vi "DisplayPathAndPose.vi"(1 "Feed Back Pointing Angle (deg)":dbl, 2 "Feed Back Distance Error (in)":dbl, 3 "Data (index by row)":dbl[][](array[numeric])) -> (0 "Path and Robot Pose":cluster{dbl[], dbl[]}[](graph))   [LabVIEW 2020]
uses:
  Globals/Sensor_Values.vi
panel:
  in  "PID Drive 2":T1(graph)
  in  "PID Heading Indicator":T1(graph)
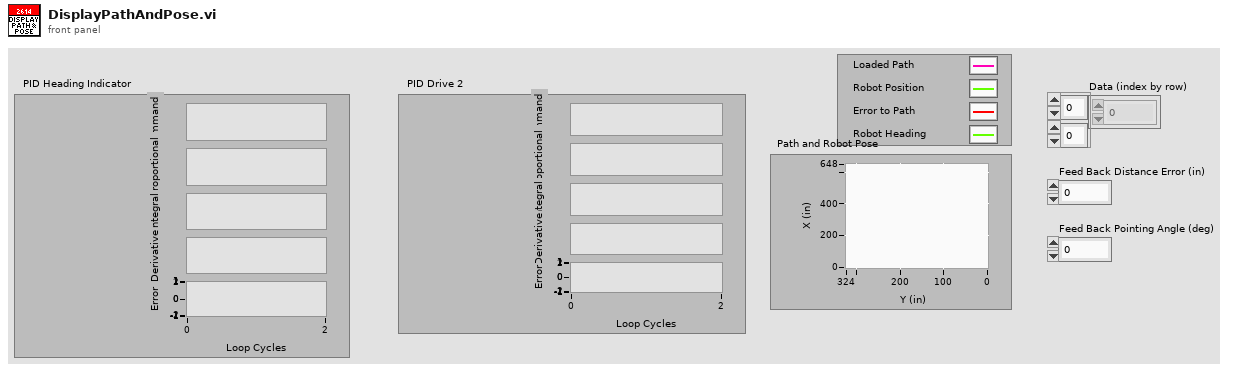
[diagram p1: front panel]
types:
  T1 = cluster{"Command":dbl, "Proportional":dbl, "Integral":dbl, "Derivative":dbl, "Goal":dbl}
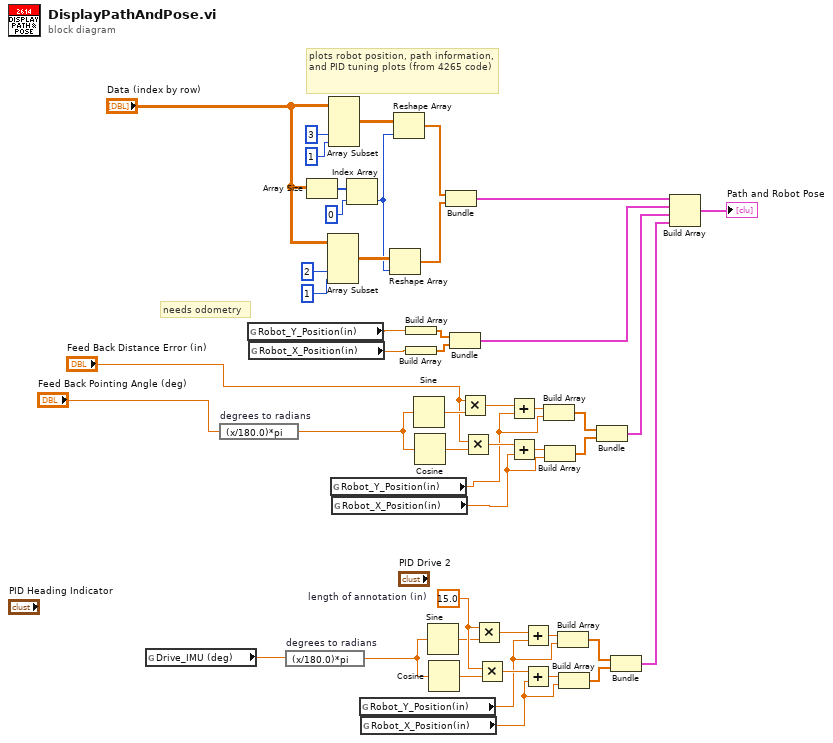
[diagram p0: block diagram]
diagram:
  w43 = 15.0  # length of annotation (in)
  # "needs odometry"
  # "plots robot position, path information, and PID tuning plots (from 4265 code)"
  n1 = global read "Sensor_Values.vi" "Drive_IMU (deg)"() -> (w7:dbl)
  n2 = expression code="(x/180.0)*pi" "degrees to radians"("Feed Back Pointing Angle (deg)") -> (w33:dbl)
  n3 = global read "Sensor_Values.vi" "Robot_Y_Position(in)"() -> (w6:dbl)
  n4 = global read "Sensor_Values.vi" "Robot_X_Position(in)"() -> (w5:dbl)
  n5 = expression code="(x/180.0)*pi" "degrees to radians"(w7) -> (w42:dbl)
  n6 = Array Size(array="Data (index by row)") -> (size(s)=w16:i32[])
  n7 = Array Subset(array="Data (index by row)", index (col)=2 ("index"), length (col)=1 ("length")) -> (w18:dbl[][])  [unwired: 2 in]
  n8 = Array Subset(array="Data (index by row)", index (col)=3 ("index"), length (col)=1 ("length")) -> (w17:dbl[][])  [unwired: 2 in]
  n9 = global read "Sensor_Values.vi" "Robot_Y_Position(in)"() -> (w4:dbl)
  n10 = global read "Sensor_Values.vi" "Robot_X_Position(in)"() -> (w3:dbl)
  n11 = Index Array(array=w16, index=0) -> (element=w15:i32)
  n12 = global read "Sensor_Values.vi" "Robot_Y_Position(in)"() -> (w2:dbl)
  n13 = global read "Sensor_Values.vi" "Robot_X_Position(in)"() -> (w1:dbl)
  n14 = Reshape Array(w18, w15) -> (w46:dbl[])
  n15 = Reshape Array(w17, w15) -> (w45:dbl[])
  n16 = Build Array(w6) -> (w9:dbl[])
  n17 = Build Array(w5) -> (w8:dbl[])
  n18 = Sine(x=w33) -> (sin(x)=w32:dbl)
  n19 = Cosine(x=w33) -> (cos(x)=w31:dbl)
  n20 = Sine(x=w42) -> (sin(x)=w41:dbl)
  n21 = Cosine(x=w42) -> (cos(x)=w40:dbl)
  n22 = Bundle(w45, w46) -> (w13:cluster{dbl[], dbl[]})  [unwired: 1 in]
  n23 = Bundle(w9, w8) -> (w24:cluster{dbl[], dbl[]})  [unwired: 1 in]
  n24 = Multiply(x="Feed Back Distance Error (in)", y=w32) -> (x*y=w30:dbl)
  n25 = Multiply(x="Feed Back Distance Error (in)", y=w31) -> (x*y=w29:dbl)
  n26 = Multiply(x=w43, y=w41) -> (x*y=w39:dbl)
  n27 = Multiply(x=w43, y=w40) -> (x*y=w38:dbl)
  n28 = Add(x=w30, y=w4) -> (x+y=w28:dbl)
  n29 = Add(x=w29, y=w3) -> (x+y=w27:dbl)
  n30 = Add(x=w39, y=w2) -> (x+y=w37:dbl)
  n31 = Add(x=w38, y=w1) -> (x+y=w36:dbl)
  n32 = Build Array(w28, w4) -> (w26:dbl[])
  n33 = Build Array(w27, w3) -> (w25:dbl[])
  n34 = Build Array(w37, w2) -> (w35:dbl[])
  n35 = Build Array(w36, w1) -> (w34:dbl[])
  n36 = Bundle(w26, w25) -> (w44:cluster{dbl[], dbl[]})  [unwired: 1 in]
  n37 = Bundle(w35, w34) -> (w47:cluster{dbl[], dbl[]})  [unwired: 1 in]
  n38 = Build Array(w13, w24, w44, w47) -> (→"Path and Robot Pose":cluster{dbl[], dbl[]}[])
